vi "Auto.vi"() -> ()   [LabVIEW 2020]
uses:
  Global_Variable/Global.vi
  Global_Variable/A180648.vi
  Global_Variable/System_Conf.vi
  Libraries/S7/S7.lvlib
panel:
  out "前序":string
  out "用户事件输出":refnum<user-event>
  out "磨合正向初始化":bool
  out "工位三开始计时1":bool
  out "产品变更_Event":refnum<user-event>
  out "T1+T2":dbl
  out "T2":dbl
  out "T1":dbl
  out "吸收电流":sgl
  out "输出扭矩(大)":sgl
  out "输入扭矩":sgl
  out "力特性逆向去程":bool
  out "力特性正向去程":bool
  out "力特性逆向回程":bool
  out "力特性正向回程":bool
  out "工位三开始计时":bool
  out "工位二开始计时":bool
  out "功能正向初始化":bool
  out "功能逆向初始化":bool
  out "空载逆向初始化":bool
  out "空载正向初始化":bool
  out "试验项目":T1(tab)
  out "压装曲线":cluster{dbl[], dbl[]}[](graph)
  out "侧铆曲线":cluster{dbl[], dbl[]}[](graph)
  out "0°曲线":cluster{dbl[], dbl[]}[](graph)
  out "45°曲线":cluster{dbl[], dbl[]}[](graph)
  out "力特性试验":cluster{dbl[], dbl[]}[](graph)
  out "功能试验":cluster{dbl[], dbl[]}[](graph)
  out "电流特性试验":cluster{dbl[], dbl[]}[](graph)
  out "逆向空载试验":cluster{dbl[], dbl[]}[](graph)
  out "磨合":cluster{dbl[], dbl[]}[](graph)
  in  "判定结果":bool[][](array[boolean])=[[TRUE]]
  in  "STEP":string
  # "车速0"
  # "车速1"
  # "车速2"
  # "车速3"
  # "车速4"
  # "车速5"
  # "车速0"
  # "车速1"
  # "车速2"
  # "车速3"
  # "车速4"
  # "车速5"
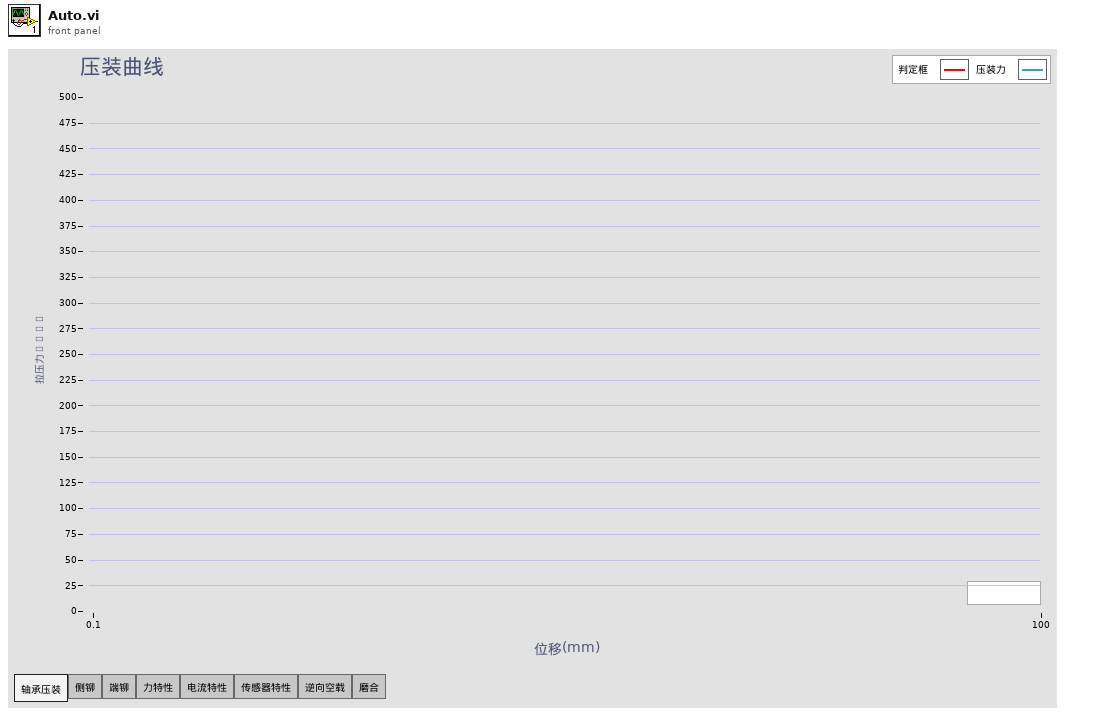
[diagram p1: front panel]
types:
  T1 = enum32{"轴承压装", "侧铆", "端铆", "力特性", "电流特性", "传感器特性", "逆向空载", "磨合"}
  T2 = enum32{"Invalid", "Standard", "Closed", "Hidden", "Minimized", "Maximized"}
  T3 = cluster{"输入轴扭矩":dbl, "输出轴扭矩小量程":dbl, "输出轴扭矩大量程":dbl}
  T4 = typedef "System_conf.ctl" = cluster{"空载滤波":bool, "逆向空载滤波":bool, "空载扭矩系数":dbl, "逆向空载扭矩系数":dbl}
  T5 = cluster{"第一段位移":cluster{"单位":string, "下限":dbl, "上限":dbl}, "第一段压力":cluster{"单位":string, "下限":dbl, "上限":dbl}, "第二段位移":cluster{"单位":string, "下限":dbl, "上限":dbl}, "第二段压力":cluster{"单位":string, "下限":dbl, "上限":dbl}}
  T6 = cluster{"第一段压力最大值":cluster{"单位":string, "下限":dbl, "上限":dbl}, "第一段压力最小值":cluster{"单位":string, "下限":dbl, "上限":dbl}, "第二段压力最大值":cluster{"单位":string, "下限":dbl, "上限":dbl}, "第二段压力最小值":cluster{"单位":string, "下限":dbl, "上限":dbl}, "最终压装位移":cluster{"单位":string, "下限":dbl, "上限":dbl}}
  T7 = typedef "lveventtype.ctl" = enum32{"Null", "Timeout", "Annotation Menu Selection", "Annotation Menu Selection?", "App Instance Close", "App Instance Close?", "Autoscale Range Change", "Bookmark Info Change", "Cell Edit", "Cell Edit?", "Cursor Grab", "Cursor Grab?", "Cursor Menu Selection", "Cursor Menu Selection?", "Cursor Move", "Cursor Release", "Data Change", "Direction Change", "Display State Change", "Drag Ended", "Drag Enter", "Drag Leave", "Drag Over", "Drag Source Update", "Drag Starting", "Drag Starting?", "Drop", "Exec State Change", "Key Down", "Key Down?", "Key Repeat", "Key Repeat?", "Key Up", "Listbox Double Click", "Menu Activation?", "Menu Selection (App)", "Menu Selection? (App)", "Menu Selection (User)", "Mouse Down", "Mouse Down?", "Mouse Enter", "Mouse Leave", "Mouse Move", "Mouse Up", "Mouse Wheel", "NI Security User Change (App)", "Pane Size", "Panel Close", "Panel Close?", "Panel Resize", "Plot Attribute Change", "Scale Range Change", "Shortcut Menu Activation?", "Shortcut Menu Selection (App)", "Shortcut Menu Selection? (App)", "Shortcut Menu Selection (User)", "Tree Double Click", "Tree Drag", "Tree Drag?", "Tree Drop", "Tree Drop?", "Tree Item Close", "Tree Item Close?", "Tree Item Open", "Tree Item Open?", "User Event", "Value Change"}
  T8 = typedef "LVPoint32TypeDef.ctl" = cluster{"Horizontal":i32, "Vertical":i32}
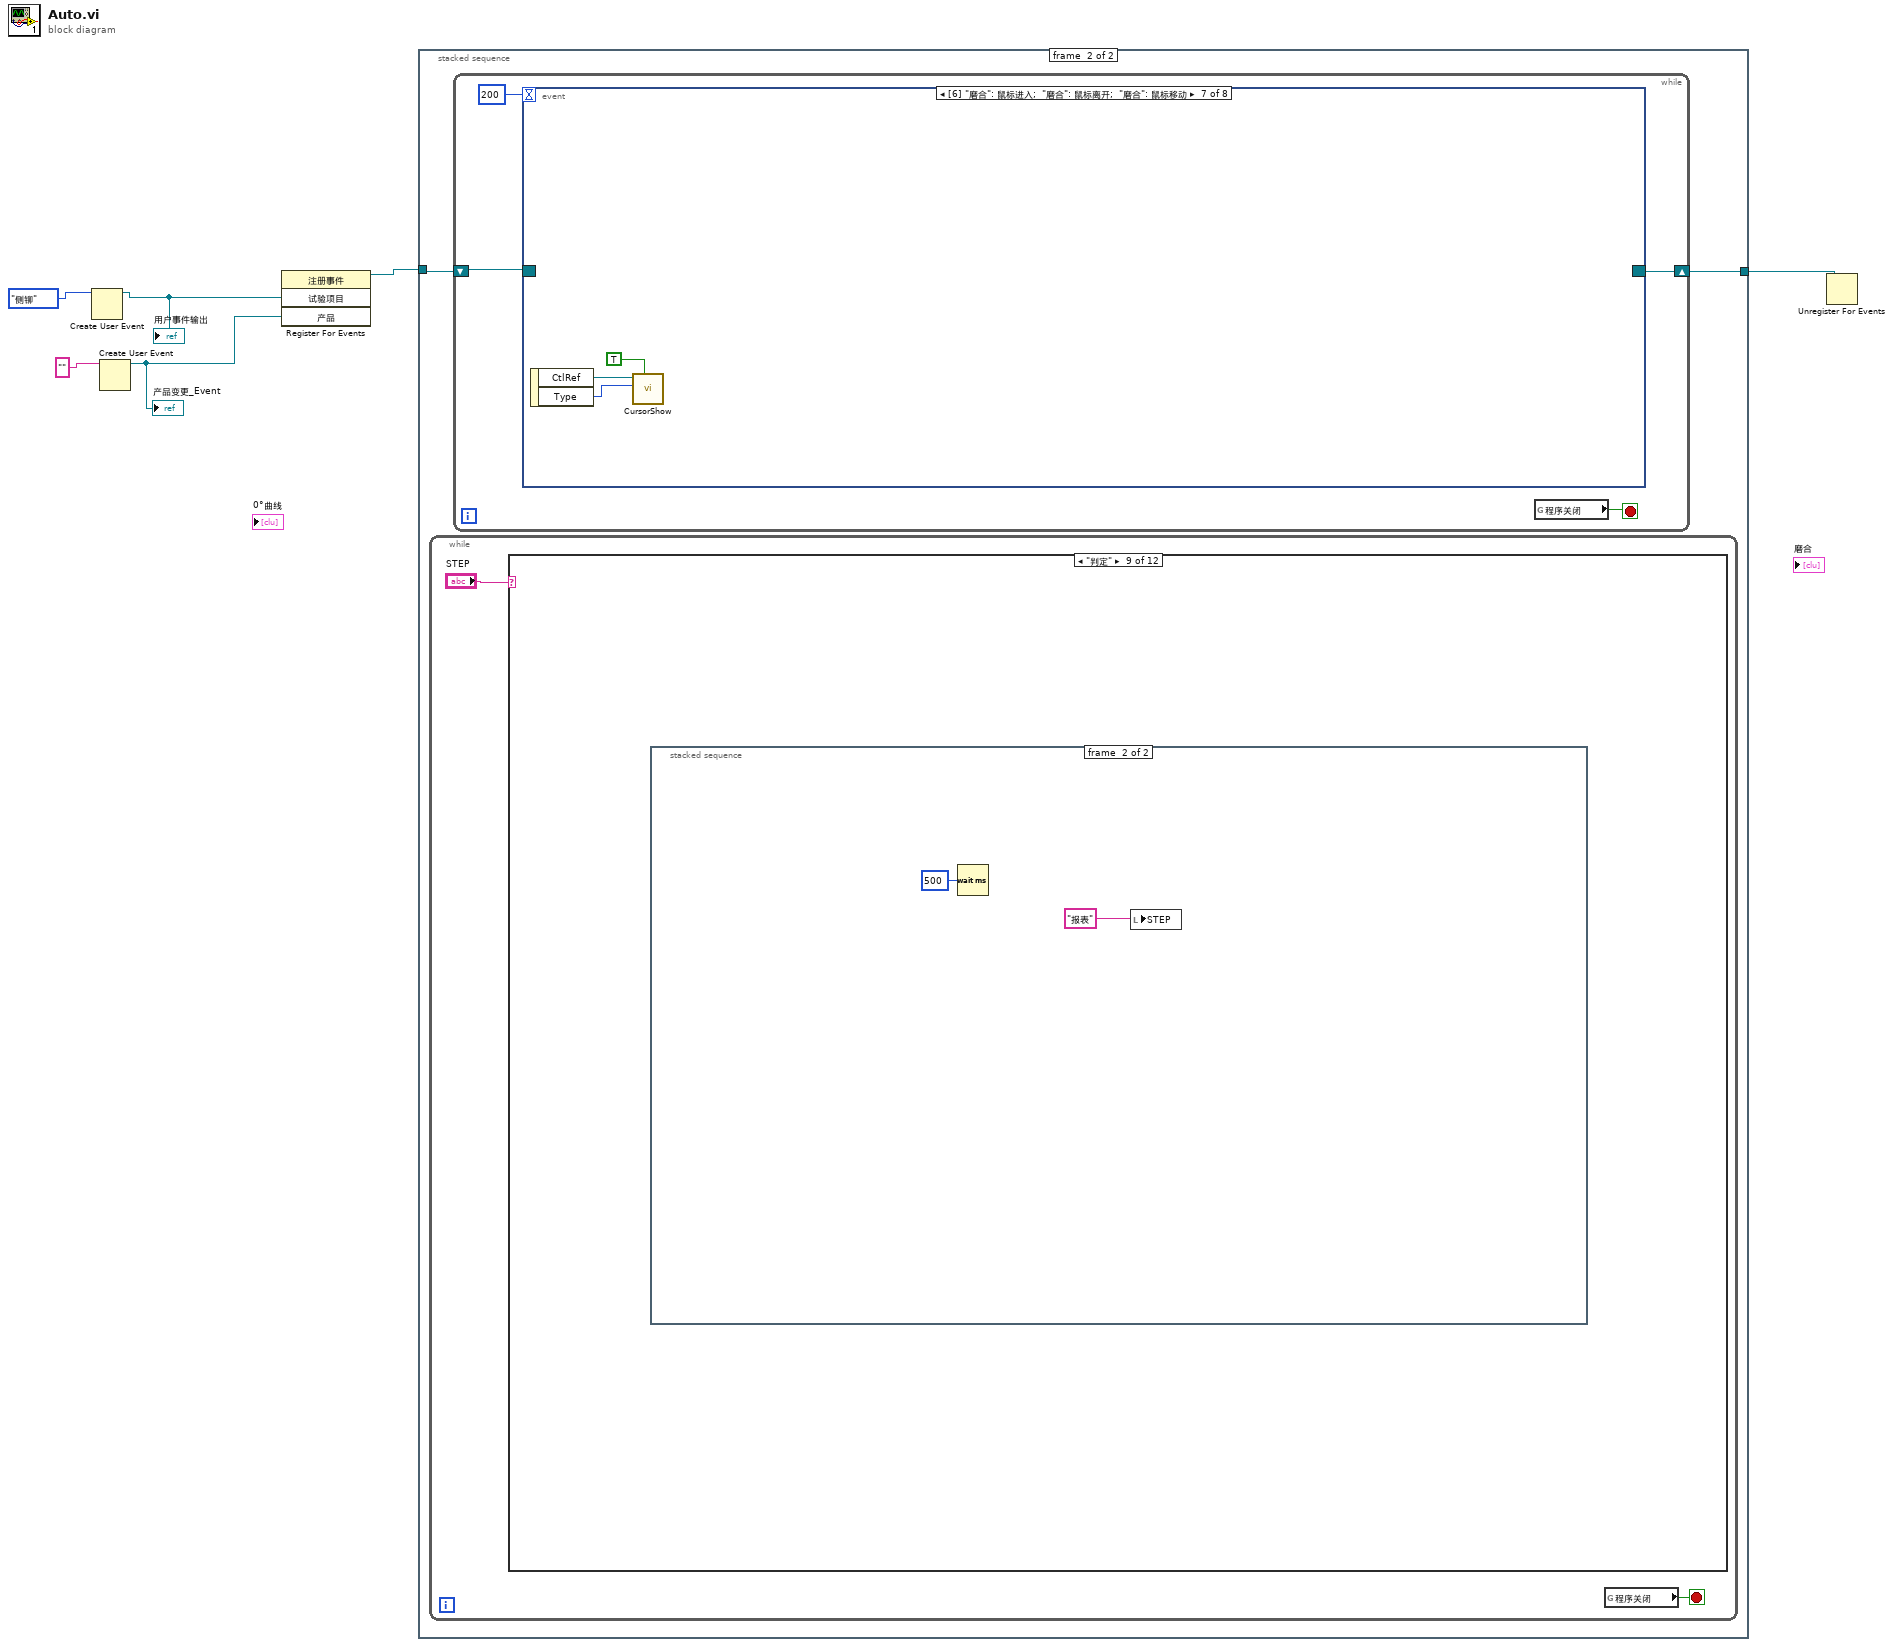
[diagram p0: block diagram]
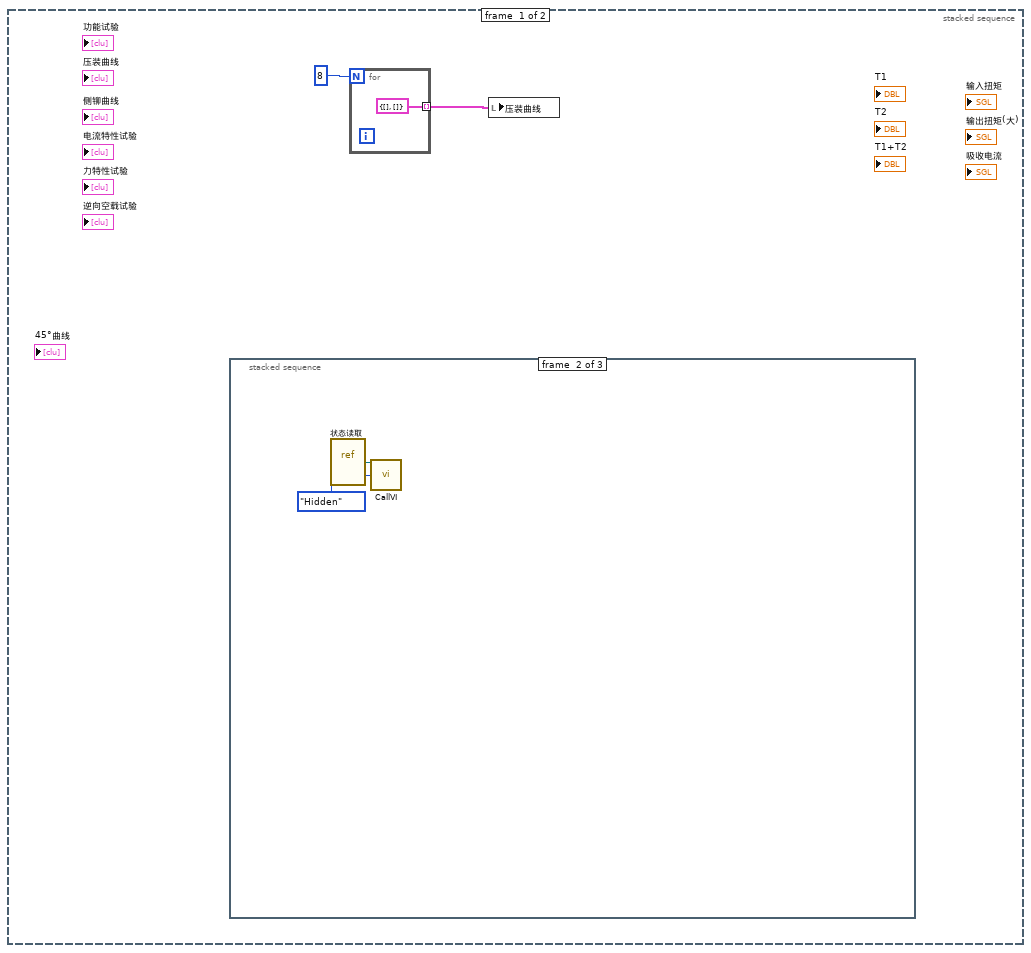
[diagram p2: hidden frame]
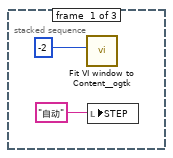
[diagram p3: hidden frame]
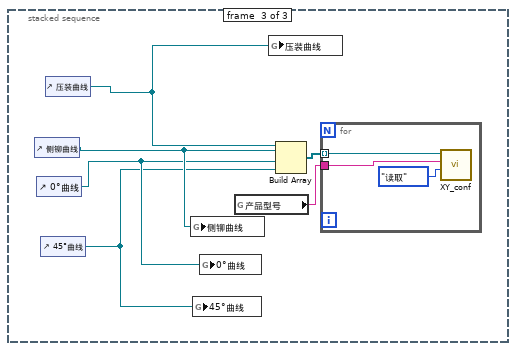
[diagram p4: hidden frame]
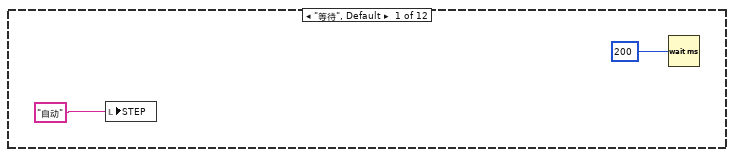
[diagram p5: hidden frame]
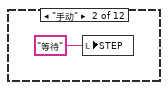
[diagram p6: hidden frame]
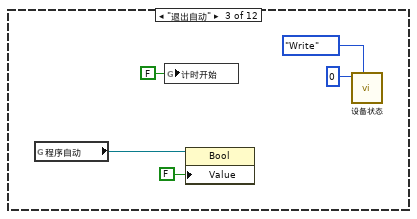
[diagram p7: hidden frame]
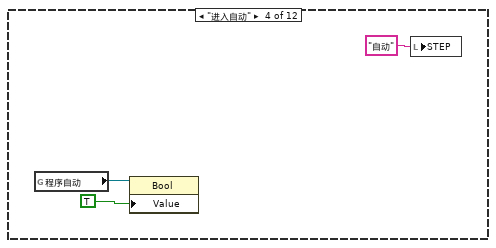
[diagram p8: hidden frame]
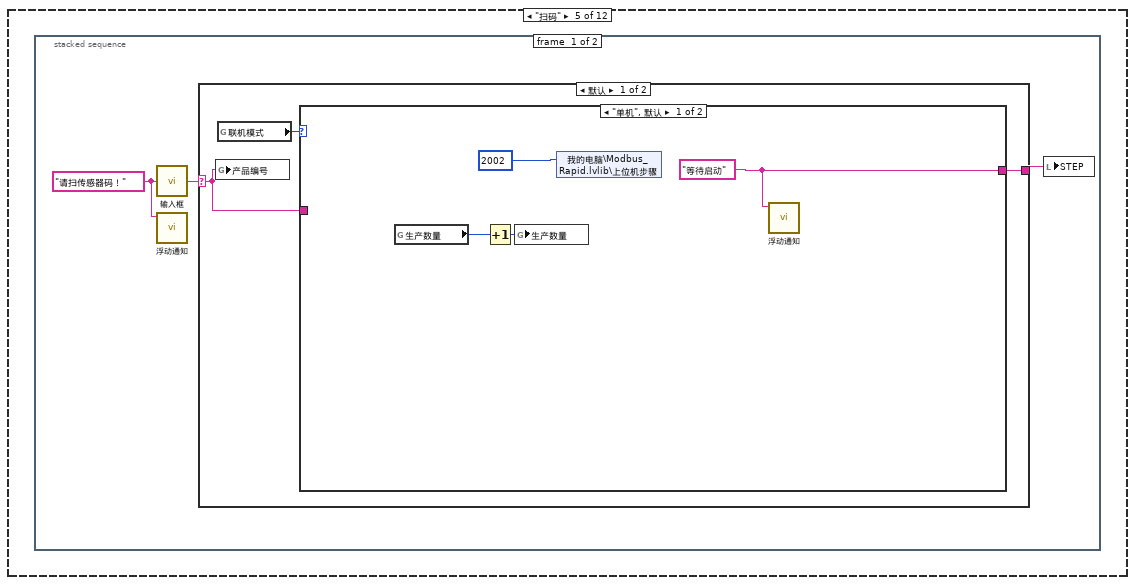
[diagram p9: hidden frame]
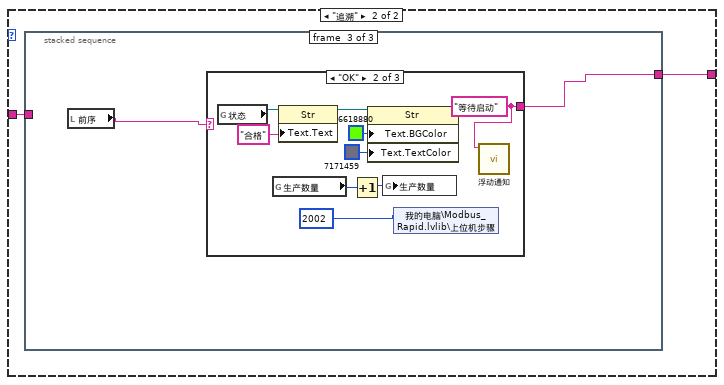
[diagram p10: hidden frame]
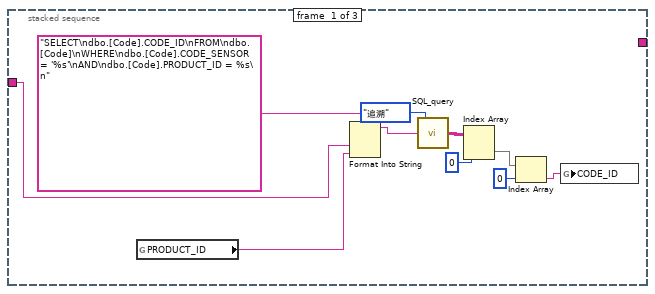
[diagram p11: hidden frame]
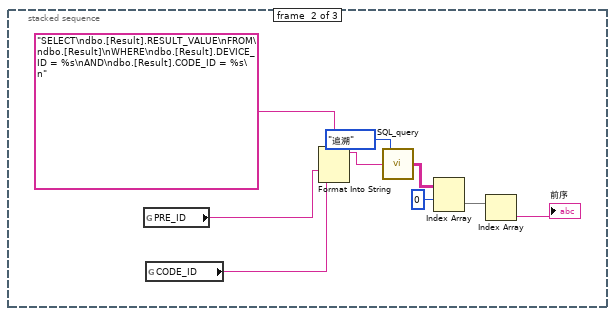
[diagram p12: hidden frame]
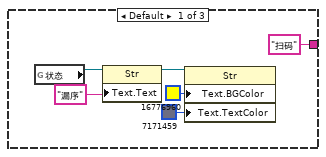
[diagram p13: hidden frame]
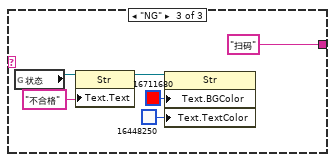
[diagram p14: hidden frame]
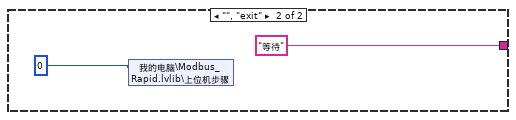
[diagram p15: hidden frame]
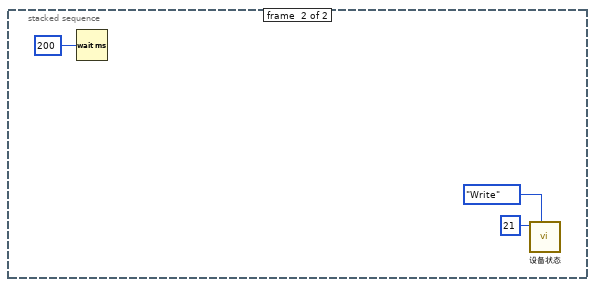
[diagram p16: hidden frame]
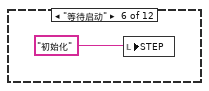
[diagram p17: hidden frame]
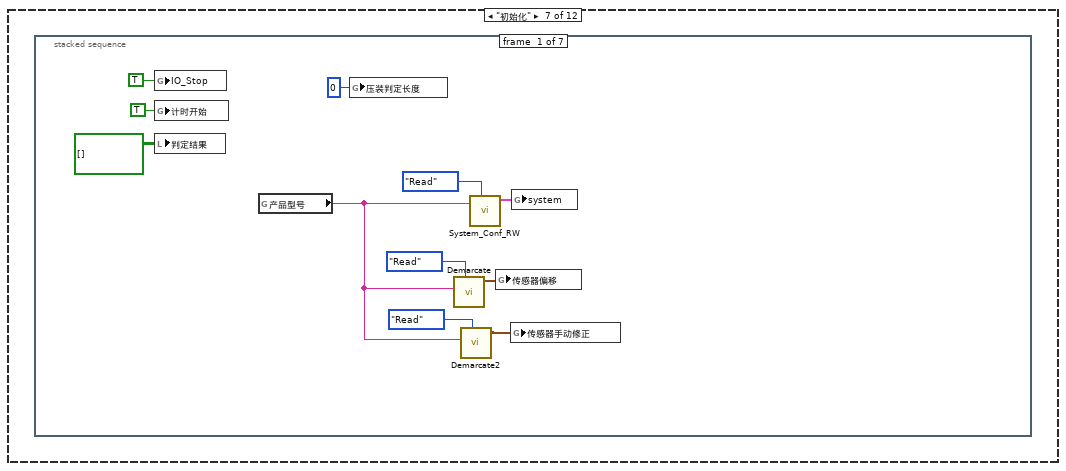
[diagram p18: hidden frame]
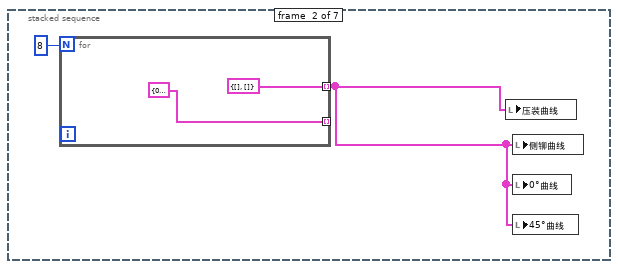
[diagram p19: hidden frame]
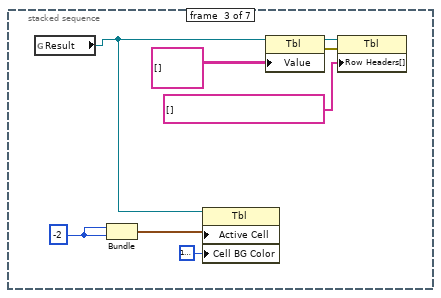
[diagram p20: hidden frame]
diagram:
  n1 = Create User Event(user event datatype=T1."侧铆" ("试验项目")) -> (user event=w1:refnum<user-event>)  [unwired: 1 in, 1 out]
  "用户事件输出" <- w1
  n2 = Create User Event(user event datatype="" ("产品")) -> (user event=w3:refnum<user-event>)  [unwired: 1 in, 1 out]
  "产品变更_Event" <- w3
  n3 = register-events(w1, w3) -> (reference out=w6:refnum<event-registration>)  [unwired: 2 in, 1 out]
  n4 = stacked-sequence {
    tunnel: w6 -> [_ w24]
    tunnel: [_ w23] -> w5
    frame #0 {
      n5 = stacked-sequence {
        frame #0 {
          n6 = call <userlib>:"Fit VI window to Content__ogtk.vi"("border spacing (2 px)"=-2) -> ()  [unwired: 5 in, 2 out]
          n7 = local write "STEP"("自动" ("STEP")) -> ()
        }
        frame #1 {
          n8 = vi-ref "状态读取.vi"() -> (w13:refnum<vi>)
          n9 = call "CallVI.vi"("VI引用"=w13, "状态"=T2."Hidden") -> ()  [unwired: 12 in, 2 out]
        }
        frame #2 {
          n10 = control-ref of="侧铆曲线"() -> (w17:refnum<vi>)
          n11 = control-ref of="0°曲线"() -> (w16:refnum<vi>)
          n12 = control-ref of="45°曲线"() -> (w15:refnum<vi>)
          n13 = control-ref of="压装曲线"() -> (w14:refnum<vi>)
          n14 = global write "A180648.vi" "侧铆曲线"(w17) -> ()
          n15 = global write "A180648.vi" "45°曲线"(w15) -> ()
          n16 = global write "A180648.vi" "0°曲线"(w16) -> ()
          n17 = global read "Global.vi" "产品型号"() -> (w18:string)
          n18 = global write "A180648.vi" "压装曲线"(w14) -> ()
          n19 = Build Array(w14, w17, w16, w15) -> (w19:refnum<vi>[])
          n20 = for {
            tunnel: w19 -> [w21] mode=indexing
            tunnel: w18 -> [w20]
            n21 = call "XY_conf.vi"("方式"=enum16{"写入", "读取"}."读取", "产品"=w20, "XY图引用"=w21) -> ()  [unwired: 4 in, 1 out]
          }
        }
      }
      n22 = for {
        N: 8 -> [_]
        tunnel: [cluster{dbl[], dbl[]} {[], []}] -> w8 mode=indexing
      }
      n23 = local write "压装曲线"(w8) -> ()
    }
    frame #1 {
      n24 = while {
        stop <- w26 stop-if-true
        n25 = case shown="\"判定\"" "STEP" {
          frame "等待", Default {
            n26 = local write "STEP"("自动" ("STEP")) -> ()
            n27 = Wait (ms)(milliseconds to wait=u32 200 ("等待时间（毫秒）")) -> ()  [unwired: 1 out]
          }
          frame "手动" {
            n28 = local write "STEP"("等待" ("STEP")) -> ()
          }
          frame "退出自动" {
            n29 = global read "Global.vi" "程序自动"() -> (w31:refnum<vi>)
            n30 = global write "Global.vi" "计时开始"(FALSE ("计时开始")) -> ()
            n31 = property class="Bool"(reference=w31, "Value"=FALSE) -> ()  [unwired: 1 in, 2 out]
            n32 = call "设备状态.vi"("枚举"=enum16{"Read", "Write"}."Write", "Status_Write"=i16 0) -> ()  [unwired: 9 in, 1 out]
          }
          frame "进入自动" {
            n33 = global read "Global.vi" "程序自动"() -> (w36:refnum<vi>)
            n34 = property class="Bool"(reference=w36, "Value"=TRUE) -> ()  [unwired: 1 in, 2 out]
            n35 = local write "STEP"("自动" ("STEP")) -> ()
          }
          frame "扫码" {
            n36 = stacked-sequence {
              frame #0 {
                w39 = "请扫传感器码！" ("提示信息")
                n37 = call "输入框.vi"("提示信息"=w39) -> ("条形码输出"=w40:string)
                n38 = call "浮动通知.vi"("通知内容"=w39) -> ()  [unwired: 11 in]
                n39 = case shown="默认" w40 {
                  selector: w40 -> [w41 _]
                  tunnel: [w43 "等待" ("State(s) in Front (\"\")")] -> w38
                  frame Default {
                    n40 = global write "Global.vi" "产品编号"(w41) -> ()
                    n41 = global read "Global.vi" "联机模式"() -> (w42:enum16{"单机", "追溯"})
                    n42 = case shown="\"单机\", 默认" w42 {
                      tunnel: [w45 w49] -> w43
                      tunnel: w41 -> [_ w48]
                      frame "单机", Default {
                        w45 = "等待启动" ("State(s) in Front (\"\")")
                        n43 = global read "Global.vi" "生产数量"() -> (w46:i32)
                        n44 = Increment(x=w46) -> (x+1=w47:i32)
                        n45 = global write "Global.vi" "生产数量"(w47) -> ()
                        n46 = shared-variable "我的电脑\\Modbus_Rapid.lvlib\\上位机步骤"(u16 2002 ("设备状态")) -> ()  [unwired: 1 in, 1 out]
                        n47 = call "浮动通知.vi"("通知内容"=w45) -> ()  [unwired: 11 in]
                      }
                      frame "追溯" {
                        n48 = stacked-sequence {
                          tunnel: [_ _ w70] -> w49
                          tunnel: w48 -> [w58 _ _]
                          frame #0 {
                            n49 = global read "追溯Global.vi" "PRODUCT_ID"() -> (w57:string)
                            n50 = Format Into String(format string="SELECT\ndbo.[Code].CODE_ID\nFROM\ndbo.[Code]\nWHERE\ndbo.[Code].CODE_SENSOR = '%s'\nAND\ndbo.[Code].PRODUCT_ID = %s\n" ("格式字符串"), w58, w57) -> (resulting string=w56:string)  [unwired: 2 in, 1 out]
                            n51 = call "SQL_query.vi"("SQL query"=w56, "联机模式"=enum16{"单机", "追溯"}."追溯") -> ("data"=w54:string[][])  [unwired: 2 in, 1 out]
                            n52 = Index Array(array=w54, index (row)=0 ("索引 (行)")) -> (element=w52:string[])  [unwired: 1 in]
                            n53 = Index Array(array=w52, index=0 ("索引")) -> (element=w50:string)
                            n54 = global write "追溯Global.vi" "CODE_ID"(w50) -> ()
                          }
                          frame #1 {
                            n55 = global read "追溯Global.vi" "PRE_ID"() -> (w67:string)
                            n56 = global read "追溯Global.vi" "CODE_ID"() -> (w66:string)
                            n57 = Format Into String(format string="SELECT\ndbo.[Result].RESULT_VALUE\nFROM\ndbo.[Result]\nWHERE\ndbo.[Result].DEVICE_ID = %s\nAND\ndbo.[Result].CODE_ID = %s\n" ("格式字符串"), w67, w66) -> (resulting string=w65:string)  [unwired: 2 in, 1 out]
                            n58 = call "SQL_query.vi"("SQL query"=w65, "联机模式"=enum16{"单机", "追溯"}."追溯") -> ("data"=w63:string[][])  [unwired: 2 in, 1 out]
                            n59 = Index Array(array=w63, index (row)=0 ("索引 (行)")) -> (element=w61:string[])  [unwired: 1 in]
                            n60 = Index Array(array=w61) -> (element=→"前序":string)  [unwired: 1 in]
                          }
                          frame #2 {
                            n61 = local read "前序"() -> (w69:string)
                            n62 = case shown="\"OK\"" w69 {
                              tunnel: ["扫码" ("State(s) in Front (\"\")") w80 "扫码" ("State(s) in Front (\"\")")] -> w70
                              frame Default {
                                n63 = global read "Global.vi" "状态"() -> (w76:refnum<vi>)
                                n64 = property class="Str"(reference=w76, "Text.Text"="漏序" ("文本.文本")) -> (reference out=w75:refnum<vi>)  [unwired: 1 in, 1 out]
                                n65 = property class="Str"(reference=w75, "Text.BGColor"=u32 16776960 ("文本.文本颜色:背景色"), "Text.TextColor"=u32 7171459 ("文本.文本颜色:文本颜色")) -> ()  [unwired: 1 in, 2 out]
                              }
                              frame "OK" {
                                w80 = "等待启动" ("State(s) in Front (\"\")")
                                n66 = global read "Global.vi" "状态"() -> (w85:refnum<vi>)
                                n67 = global read "Global.vi" "生产数量"() -> (w78:i32)
                                n68 = property class="Str"(reference=w85, "Text.Text"="合格" ("文本.文本")) -> (reference out=w83:refnum<vi>)  [unwired: 1 in, 1 out]
                                n69 = Increment(x=w78) -> (x+1=w79:i32)
                                n70 = property class="Str"(reference=w83, "Text.BGColor"=u32 6618880 ("文本.文本颜色:背景色"), "Text.TextColor"=u32 7171459 ("文本.文本颜色:文本颜色")) -> ()  [unwired: 1 in, 2 out]
                                n71 = global write "Global.vi" "生产数量"(w79) -> ()
                                n72 = shared-variable "我的电脑\\Modbus_Rapid.lvlib\\上位机步骤"(u16 2002 ("设备状态")) -> ()  [unwired: 1 in, 1 out]
                                n73 = call "浮动通知.vi"("通知内容"=w80) -> ()  [unwired: 11 in]
                              }
                              frame "NG" {
                                n74 = global read "Global.vi" "状态"() -> (w91:refnum<vi>)
                                n75 = property class="Str"(reference=w91, "Text.Text"="不合格" ("文本.文本")) -> (reference out=w89:refnum<vi>)  [unwired: 1 in, 1 out]
                                n76 = property class="Str"(reference=w89, "Text.BGColor"=u32 16711680 ("文本.文本颜色:背景色"), "Text.TextColor"=u32 16448250 ("文本.文本颜色:文本颜色")) -> ()  [unwired: 1 in, 2 out]
                              }
                            }
                          }
                        }
                      }
                    }
                  }
                  frame "", "exit" {
                    n77 = shared-variable "我的电脑\\Modbus_Rapid.lvlib\\上位机步骤"(u16 0 ("设备状态")) -> ()  [unwired: 1 in, 1 out]
                  }
                }
                n78 = local write "STEP"(w38) -> ()
              }
              frame #1 {
                n79 = Wait (ms)(milliseconds to wait=u32 200 ("等待时间（毫秒）")) -> ()  [unwired: 1 out]
                n80 = call "设备状态.vi"("枚举"=enum16{"Read", "Write"}."Write", "Status_Write"=i16 21) -> ()  [unwired: 9 in, 1 out]
              }
            }
          }
          frame "等待启动" {
            n81 = local write "STEP"("初始化" ("STEP")) -> ()
          }
          frame "初始化" {
            n82 = stacked-sequence {
              frame #0 {
                n83 = global write "Global.vi" "IO_Stop"(TRUE ("IO_Stop")) -> ()
                n84 = global write "Global.vi" "计时开始"(TRUE ("计时开始")) -> ()
                n85 = local write "判定结果"(bool[][] [] ("判定结果")) -> ()
                n86 = global read "Global.vi" "产品型号"() -> (w99:string)
                n87 = global write "判定参数.vi" "压装判定长度"(0 ("拉轴判定长度")) -> ()
                n88 = call "Demarcate.vi"("Mode"=enum16{"Read", "Write"}."Read", "Section"=w99) -> ("Sensor OUT"=w103:T3)  [unwired: 8 in, 1 out]
                n89 = call "Demarcate2.vi"("Mode"=enum16{"Read", "Write"}."Read", "Section"=w99) -> ("Sensor OUT"=w102:T3)  [unwired: 8 in, 1 out]
                n90 = call "System_Conf_RW.vi"("Mode"=enum16{"Read", "Write"}."Read", "Section"=w99) -> ("system_out"=w105:T4)  [unwired: 8 in, 1 out]
                n91 = global write "传感器偏移.vi" "传感器偏移"(w103) -> ()
                n92 = global write "传感器偏移.vi" "传感器手动修正"(w102) -> ()
                n93 = global write "System_Conf.vi" "system"(w105) -> ()
              }
              frame #1 {
                n94 = for {
                  N: 8 -> [_]
                  tunnel: [cluster{dbl[], dbl[]} {[], []}] -> w109 mode=indexing
                  tunnel: [cluster{"f0":dbl, "df":dbl, "magnitude":dbl[]} {"f0"=0.0, "df"=0.0, "magnitude"=[]} ("power spectrum [dB EU]")] -> _ mode=indexing
                }
                n95 = local write "压装曲线"(w109) -> ()
                n96 = local write "侧铆曲线"(w109) -> ()
                n97 = local write "0°曲线"(w109) -> ()
                n98 = local write "45°曲线"(w109) -> ()
              }
              frame #2 {
                w114 = -2
                n99 = global read "Global.vi" "Result"() -> (w116:refnum<vi>)
                n100 = Bundle(w114, w114) -> (w113:cluster{i32, i32})  [unwired: 1 in]
                n101 = property class="Tbl"(reference=w116, "Active Cell"=w113, "Cell BG Color"=u32 16777216 ("活动单元格:单元格背景色")) -> ()  [unwired: 1 in, 2 out]
                n102 = property class="Tbl"(reference=w116, "Value"=string[][] []) -> (reference out=w119:refnum<vi>, error out=w120:errorcluster)  [unwired: 1 in]
                n103 = property class="Tbl"(reference=w119, error in=w120, "Row Headers[]"=string[] [] ("列首字符串[]")) -> ()  [unwired: 2 out]
              }
              frame #3 {
                n104 = global read "A180648.vi" "LED-轴承压装"() -> (w124:refnum<vi>)
                n105 = global read "A180648.vi" "LED-端铆"() -> (w121:refnum<vi>)
                n106 = global read "A180648.vi" "LED-侧铆"() -> (w122:refnum<vi>)
                n107 = Build Array(w124, w122, w121) -> (w123:refnum<vi>[])
                n108 = for {
                  tunnel: w123 -> [w125] mode=indexing
                  n109 = property class="Bool"(reference=w125, "Colors [4]"=cluster{u32, u32}[] [{12369084, 12369084}] ("颜色[4]")) -> ()  [unwired: 1 in, 2 out]
                }
              }
              frame #4 {
                w128 = 1 ("维数大小")
                n110 = Initialize Array(" " ("字符串"), w128, w128, w128) -> (w130:string[][][])
                n111 = global write "A180648.vi" "当前检测项"(enum32{"拉轴", "卡簧", "完成"}."拉轴" ("当前检测项")) -> ()
                n112 = global write "A180648.vi" "检测结果"(w130) -> ()
              }
              frame #5 {
                n113 = local read "压装曲线"() -> (w132:cluster{dbl[], dbl[]}[])
                n114 = global read "判定参数.vi" "判定框"() -> (w133:T5)
                n115 = for {
                  tunnel: w132 -> [w136] mode=indexing
                  tunnel: [w135] -> w131 mode=indexing
                  tunnel: w133 -> [w134]
                  i -> [w137]
                  n116 = case shown="0" w137 {
                    tunnel: w136 -> [w138 _]
                    tunnel: [w138 w141] -> w135
                    tunnel: w134 -> [_ w146]
                    frame Default {
                    }
                    frame 0 {
                      n117 = Unbundle By Name(w146) -> ("第一段位移.下限"=w145:dbl, "第一段位移.上限"=w144:dbl, "第一段压力.下限"=w139:dbl, "第一段压力.上限"=w140:dbl)
                      n118 = Build Array(w144, w144, w145, w145, w144) -> (w143:dbl[])
                      n119 = Build Array(w139, w140, w140, w139, w139) -> (w142:dbl[])
                      n120 = Bundle(w143, w142) -> (w141:cluster{dbl[], dbl[]})  [unwired: 1 in]
                    }
                  }
                }
                n121 = local write "压装曲线"(w131) -> ()
              }
              frame #6 {
                w148 = TRUE
                n122 = local write "STEP"("自动" ("STEP")) -> ()
                "工位三开始计时" <- w148
                "工位二开始计时" <- w148
                "空载正向初始化" <- w148
                "空载逆向初始化" <- w148
                "功能正向初始化" <- w148
                "功能逆向初始化" <- w148
                "力特性逆向去程" <- w148
                "力特性正向去程" <- w148
                "力特性逆向回程" <- w148
                "力特性正向回程" <- w148
                "磨合正向初始化" <- w148
                "工位三开始计时1" <- w148
              }
            }
          }
          frame "试验项" {
            n123 = global read "A180648.vi" "当前检测项"() -> (w149:enum32{"拉轴", "卡簧", "完成"})
            n124 = case shown="\"拉轴\", 默认" w149 {
              selector: w149 -> [w151 _]
              tunnel: [w154 "报表" ("STEP")] -> w150
              frame "拉轴", Default {
                n125 = global read "Global.vi" "试验项目"() -> (w152:bool[])
                n126 = Index Array(array=w152, index=w151) -> (element=w153:bool)
                n127 = case shown="真" w153 {
                  tunnel: ["试验项" ("字符串") w161] -> w154
                  tunnel: w151 -> [_ w162]
                  frame False {
                    n128 = global read "A180648.vi" "当前检测项"() -> (w159:enum32{"拉轴", "卡簧", "完成"})
                    n129 = Increment(x=w159) -> (x+1=w158:enum32{"拉轴", "卡簧", "完成"})
                    n130 = global write "A180648.vi" "当前检测项"(w158) -> ()
                    n131 = local read "判定结果"() -> (w155:bool[][])
                    n132 = Build Array (concatenate)(w155, bool[] [FALSE] ("判定结果")) -> (w156:bool[][])
                    n133 = local write "判定结果"(w156) -> ()
                  }
                  frame True {
                    n134 = case shown="\"拉轴\", 默认" w162 {
                      tunnel: ["等待" ("STEP") "等待" ("STEP") "报表" ("STEP")] -> w161
                      frame "拉轴", Default {
                        n135 = call "浮动通知.vi"("通知内容"="拉拔力试验") -> ()  [unwired: 11 in]
                        n136 = property on="试验项目" class="TabCtl (严格)"("Val(Sgnl)"=T1."轴承压装" ("值(信号)")) -> ()  [unwired: 2 in, 2 out]
                      }
                      frame "卡簧" {
                        n137 = call "浮动通知.vi"("通知内容"="卡簧检测") -> ()  [unwired: 11 in]
                      }
                      frame "完成" {
                      }
                    }
                  }
                }
              }
              frame "完成" {
              }
            }
            n138 = local write "STEP"(w150) -> ()
          }
          frame "判定" {
            n139 = stacked-sequence {
              frame #0 {
                n140 = global read "判定参数.vi" "压装判定参数"() -> (w181:T6)
                n141 = local read "压装曲线"() -> (w182:cluster{dbl[], dbl[]}[])
                n142 = global read "Global.vi" "Result"() -> (w180:refnum<vi>)
                n143 = call "压装试验判定.vi"("Result"=w180, "判定参数"=w181, "XY曲线"=w182) -> ("判定项长度"=w171:i32, "OK？"=w170:bool)  [unwired: 7 in]
                n144 = global read "A180648.vi" "LED-轴承压装"() -> (w176:refnum<vi>)
                n145 = local read "判定结果"() -> (w172:bool[][])
                n146 = Select(t=cluster{u32, u32}[] [{6618880, 6618880}, {6618880, 6618880}, {6618880, 6618880}, {6618880, 6618880}] ("颜色[4]"), s=w170, f=cluster{u32, u32}[] [{16711680, 16711680}, {16711680, 16711680}, {16711680, 16711680}, {16711680, 16711680}] ("颜色[4]")) -> (s? t:f=w177:cluster{u32, u32}[])
                n147 = Build Array(TRUE, w170) -> (w175:bool[])
                n148 = global write "判定参数.vi" "压装判定长度"(w171) -> ()
                n149 = property class="Bool"(reference=w176, "Colors [4]"=w177) -> ()  [unwired: 1 in, 2 out]
                n150 = Build Array (concatenate)(w172, w175) -> (w173:bool[][])
                n151 = case shown="真" w170 {
                  frame False {
                    n152 = shared-variable "我的电脑\\Modbus_Rapid.lvlib\\工位1合格状态"(u16 2 ("工位1合格状态")) -> ()  [unwired: 1 in, 1 out]
                  }
                  frame True {
                    n153 = shared-variable "我的电脑\\Modbus_Rapid.lvlib\\工位1合格状态"(u16 1 ("工位1合格状态")) -> ()  [unwired: 1 in, 1 out]
                  }
                }
                n154 = local write "判定结果"(w173) -> ()
              }
              frame #1 {
                n155 = Wait (ms)(milliseconds to wait=u32 500 ("等待时间（毫秒）")) -> ()  [unwired: 1 out]
                n156 = local write "STEP"("报表") -> ()
              }
            }
          }
          frame "自动" {
            n157 = shared-variable "我的电脑\\Modbus_Rapid.lvlib\\上位机步骤"() -> (w187:u16)  [unwired: 1 in, 1 out]
            n158 = case shown="10" w187 {
              frame 127 {
                n159 = global write "Global.vi" "计时开始"(FALSE ("计时开始")) -> ()
                n160 = call "浮动通知.vi"("通知内容"="复位中……" ("Status")) -> ()  [unwired: 11 in]
              }
              frame 128 {
                n161 = call "浮动通知.vi"("通知内容"="复位完成" ("Status")) -> ()  [unwired: 11 in]
              }
              frame Default {
              }
              frame 0 {
                n162 = disable-structure shown="禁用" {
                  frame Disabled {
                    n163 = global write "Global.vi" "计时开始"(FALSE ("计时开始")) -> ()
                  }
                  frame Enabled {
                  }
                }
              }
              frame 2 {
                n164 = local write "STEP"("初始化" ("STEP")) -> ()
              }
              frame 5 {
                n165 = shared-variable "我的电脑\\Modbus_Rapid.lvlib\\上位机步骤"(u16 10 ("上位机状态")) -> ()  [unwired: 1 in, 1 out]
              }
              frame 7 {
                n166 = shared-variable "我的电脑\\Modbus_Rapid.lvlib\\电缸参数"() -> (w197:sgl[])  [unwired: 1 in, 1 out]
                n167 = disable-structure shown="禁用" {
                  frame Disabled {
                    n168 = local read "压装曲线"() -> (w200:cluster{dbl[], dbl[]}[])
                    n169 = for {
                      tunnel: [w202] -> _ mode=indexing
                      tunnel: w200 -> [w201] mode=indexing
                      i -> [w203]
                      n170 = case shown="2" w203 {
                        tunnel: [_ w204] -> w202
                        tunnel: w201 -> [_ w209]
                        frame Default {
                        }
                        frame 2 {
                          n171 = Unbundle(w209) -> (w208:dbl[], w207:dbl[])
                          n172 = Build Array(w208) -> (w206:dbl[][])  [unwired: 1 in]
                          n173 = Build Array(w207) -> (w205:dbl[][])  [unwired: 1 in]
                          n174 = Bundle(w206, w205) -> (w204:cluster{dbl[][], dbl[][]})  [unwired: 1 in]
                        }
                      }
                    }
                    n175 = local read "压装曲线"() -> ()  [unwired: 1 in]
                  }
                  frame Enabled {
                  }
                }
                n176 = Index Array(array=w197, index=1 ("索引")) -> (element=w196:sgl)
                n177 = Index Array(array=w197) -> (element=w195:sgl)  [unwired: 1 in]
                n178 = control-ref of="压装曲线"() -> (w199:refnum<vi>)
                n179 = call "曲线采集.vi"("曲线引用"=w199, "曲线索引"=2, "X"=w196, "Y"=w195) -> ()  [unwired: 10 in, 2 out]
              }
              frame 8 {
                n180 = call "浮动通知.vi"("通知内容"="程序停止！" ("Status")) -> ()  [unwired: 11 in]
              }
              frame 10 {
                n181 = local write "STEP"("判定" ("STEP")) -> ()
              }
              frame 20 {
                n182 = shared-variable "我的电脑\\Modbus_Rapid.lvlib\\上位机步骤"() -> (w212:u16)  [unwired: 1 in, 1 out]
                n183 = case shown="2000" w212 {
                  frame 0, Default {
                  }
                  frame 2000 {
                    n184 = local write "STEP"("扫码" ("STEP")) -> ()
                  }
                }
              }
              frame 100 {
                n185 = call "浮动通知.vi"("通知内容"="请安装工件到位启动！" ("Status")) -> ()  [unwired: 11 in]
              }
              frame 105 {
                n186 = call "浮动通知.vi"("通知内容"="压紧缸下降！" ("Status")) -> ()  [unwired: 11 in]
              }
              frame 120 {
                n187 = call "浮动通知.vi"("通知内容"="夹爪夹紧！" ("Status")) -> ()  [unwired: 11 in]
              }
              frame 130 {
                n188 = call "浮动通知.vi"("通知内容"="拉升磨合" ("Status")) -> ()  [unwired: 11 in]
              }
              frame 161 {
                n189 = call "浮动通知.vi"("通知内容"="夹爪松开" ("Status")) -> ()  [unwired: 11 in]
                n190 = local write "STEP"("判定" ("STEP")) -> ()
              }
              frame 163 {
                n191 = call "浮动通知.vi"("通知内容"="请取记号笔" ("Status")) -> ()  [unwired: 11 in]
              }
              frame 999 {
                n192 = call "浮动通知.vi"("通知内容"="请启动！" ("Status")) -> ()  [unwired: 11 in]
              }
              frame 2000 {
                n193 = shared-variable "我的电脑\\Modbus_Rapid.lvlib\\上位机步骤"(u16 2001 ("上位机步骤")) -> ()  [unwired: 1 in, 1 out]
                n194 = local write "STEP"("扫码" ("STEP")) -> ()
              }
              frame 1002 {
              }
              frame 1024 {
                n195 = local write "STEP"("退出自动" ("STEP")) -> ()
              }
            }
          }
          frame "合格判定" {
            n196 = Wait (ms)(milliseconds to wait=u32 100 ("等待时间（毫秒）")) -> ()  [unwired: 1 out]
            n197 = local write "STEP"("等待" ("STEP")) -> ()
          }
          frame "报表" {
            n198 = stacked-sequence {
              seq-local: [_ w231 _ _] -> [_ _ w236 _]
              frame #0 {
                n199 = global write "Global.vi" "计时开始"(FALSE ("计时开始")) -> ()
                n200 = disable-structure shown="禁用" {
                  frame Disabled {
                    n201 = global read "Global.vi" "产品编号"() -> (w230:string)
                    n202 = call "Get_CODE_ID.vi"("CODE_MAIN"=w230) -> ("CODE_ID"=w229:string)  [unwired: 10 in]
                    n203 = global write "追溯Global.vi" "CODE_ID"(w229) -> ()
                  }
                  frame Enabled {
                  }
                }
                n204 = shared-variable "我的电脑\\Modbus_Rapid.lvlib\\上位机步骤"(u16 1000 ("上位机状态")) -> ()  [unwired: 1 in, 1 out]
              }
              frame #1 {
                n205 = global read "Global.vi" "产品编号"() -> (w232:string)
                n206 = call "Report.vi"("文件重命名"=TRUE, "文件名称"=w232, "检测结果"="判定结果") -> ("PRODUCT_VAULE"=w231:string)  [unwired: 7 in, 1 out]
              }
              frame #2 {
                n207 = global read "Global.vi" "联机模式"() -> (w235:enum16{"单机", "追溯"})
                n208 = case shown="\"追溯\"" w235 {
                  tunnel: w236 -> [_ w237]
                  frame "单机", Default {
                  }
                  frame "追溯" {
                    n209 = global read "Global.vi" "Result"() -> (w239:refnum<vi>)
                    n210 = property class="Tbl"(reference=w239) -> (reference out=w244:refnum<vi>, error out=w241:errorcluster, "Row Headers[]"=w242:string[])  [unwired: 1 in]
                    n211 = property class="Tbl"(reference=w244, error in=w241) -> (error out=w240:errorcluster, "Value"=w243:string[][])  [unwired: 1 out]
                    n212 = for {
                      tunnel: w243 -> [w251] mode=indexing
                      tunnel: w242 -> [w252] mode=indexing
                      tunnel: [w249] -> w238 mode=indexing if=w250
                      shift-right: [w248] -> _
                      shift-left: w240 -> [w248]
                      n213 = Build Array (concatenate)(w252, w251) -> (w249:string[])
                      n214 = Index Array(array=w251) -> (element=w253:string)  [unwired: 1 in]
                      n215 = case shown="\"\"" w253 {
                        tunnel: [TRUE FALSE] -> w250
                        frame Default {
                        }
                        frame "" {
                        }
                      }
                    }
                    n216 = global read "追溯Global.vi" "DEVICE_ID"() -> (w246:string)
                    n217 = global read "追溯Global.vi" "CODE_ID"() -> (w247:string)
                    n218 = global read "追溯Global.vi" "USER_ID"() -> (w245:string)
                    n219 = call "UPTEST.vi"("Result"=w238, "CODE_ID"=w247, "DEVICE_ID"=w246) -> ()  [unwired: 6 in, 1 out]
                    n220 = call "UPRESULT.vi"("DEVICE_ID"=w246, "USER_ID"=w245, "CODE_ID"=w247, "RESULT_VALUE"=w237) -> ()  [unwired: 11 in, 1 out]
                  }
                }
              }
              frame #3 {
                n221 = global read "检测结果.vi" "合格状态"() -> (w257:string)
                n222 = local write "STEP"("进入自动" ("STEP")) -> ()
                n223 = case shown="\"假\", 默认" w257 {
                  frame "假", Default {
                  }
                  frame "合格" {
                    n224 = global read "Global.vi" "合格数量"() -> (w260:i32)
                    n225 = Increment(x=w260) -> (x+1=w259:i32)
                    n226 = global write "Global.vi" "合格数量"(w259) -> ()
                  }
                }
                n227 = Wait (ms)(milliseconds to wait=u32 1000 ("等待时间（毫秒）")) -> ()  [unwired: 1 out]
              }
            }
          }
        }
        n228 = global read "Global.vi" "程序关闭"() -> (w26:bool)
      }
      n229 = while {
        shift-right: [w261] -> w23
        shift-left: w24 -> [w262]
        stop <- w263 stop-if-true
        n230 = event shown="[6] \"磨合\": 鼠标进入;  \"磨合\": 鼠标离开;  \"磨合\": 鼠标移动" {
          selector: w262 -> [_ _ _ _ _ _ _ _]
          dyn-events: [_ _ _ _ _ _ _ _] -> w261
          timeout: 200 -> [_ _ _ _ _ _ _ _]
          event Timeout {
            n231 = event-data() -> ()  [unwired: 1 in, 3 out]
            n232 = call "Obtain Broadcast Events for Registration.vi"() -> ("Already running?"=w265:bool)  [unwired: 9 in, 2 out]
            n233 = case shown="真" w265 {
              frame False {
                n234 = local write "STEP"("手动" ("STEP")) -> ()
              }
              frame True {
                n235 = call "错误代码.vi"() -> ("Status_Read"=w267:u32)  [unwired: 11 in]
                n236 = feedback #1() -> (w277:u32)  [unwired: 1 in]
                n237 = feedback-in #1(w267) -> ()
                n238 = case shown="0" w267 {
                  frame 0 {
                    n239 = global read "Global.vi" "报警图标"() -> (w278:refnum<vi>)
                    n240 = property class="Bool"(reference=w278, "Visible"=FALSE ("可见")) -> ()  [unwired: 1 in, 2 out]
                  }
                  frame 1, Default {
                    n241 = global read "Global.vi" "报警图标"() -> (w281:refnum<vi>)
                    n242 = property class="Bool"(reference=w281, "Visible"=TRUE ("可见")) -> ()  [unwired: 1 in, 2 out]
                  }
                }
                n243 = Greater Or Equal?(x=w267, y=i16 5000) -> (x >= y?=w275:bool)
                n244 = Less?(x=w267, y=i16 5200) -> (x < y?=w276:bool)
                n245 = Equal?(x=w267, y=w277) -> (x = y?=w274:bool)
                n246 = global read "Global.vi" "报警图标"() -> (w269:refnum<vi>)
                n247 = And(x=w275, y=w276) -> (x .and. y?=w268:bool)
                n248 = property class="Bool"(reference=w269, "Value"=w268) -> ()  [unwired: 1 in, 2 out]
                n249 = Bundle By Name(cluster=errorcluster {"status"=FALSE, "code"=0, "source"=""} ("错误常量"), "status"=w268, "code"=w267) -> (w273:errorcluster)
                n250 = case shown="假" w274 {
                  tunnel: w273 -> [w282 _]
                  frame False {
                    n251 = call "报警处理.vi"("错误常量"=w282) -> ()  [unwired: 9 in, 2 out]
                  }
                  frame True {
                  }
                }
              }
            }
          }
          event User Event {
            n252 = event-data() -> ("试验项目"=w283:T1)  [unwired: 1 in]
            "试验项目" <- w283
            n253 = disable-structure shown="禁用" {
              disable-tunnel: w283 -> [w284 _]
              frame Disabled {
                n254 = global read "A180648.vi" "检测结果"() -> (w287:string[][][])
                n255 = global read "Global.vi" "Result"() -> (w285:refnum<vi>)
                n256 = Index Array(array=w287, index (dim 0)=w284) -> (element=w286:string[][])  [unwired: 2 in]
                n257 = property class="Tbl"(reference=w285, "Value"=w286) -> ()  [unwired: 1 in, 2 out]
              }
              frame Enabled {
              }
            }
          }
          event "试验项目": Value Change {
            n258 = event-data() -> ("NewVal"=w288:T1)  [unwired: 1 in]
            n259 = disable-structure shown="禁用" {
              disable-tunnel: w288 -> [w292 _]
              frame Disabled {
                n260 = global read "A180648.vi" "检测结果"() -> (w291:string[][][])
                n261 = global read "Global.vi" "Result"() -> (w289:refnum<vi>)
                n262 = Index Array(array=w291, index (dim 0)=w292) -> (element=w290:string[][])  [unwired: 2 in]
                n263 = property class="Tbl"(reference=w289, "Value"=w290) -> ()  [unwired: 1 in, 2 out]
              }
              frame Enabled {
              }
            }
          }
          event "0°曲线", "侧铆曲线", "45°曲线", "压装曲线", "功能试验", "逆向空载试验", "磨合": Scale Range Change {
            n264 = event-data() -> ("CtlRef"=w294:refnum<vi>)  [unwired: 1 in, 4 out]
            n265 = global read "Global.vi" "产品型号"() -> (w293:string)
            n266 = call "XY_conf.vi"("方式"=enum16{"写入", "读取"}."写入", "产品"=w293, "XY图引用"=w294) -> ()  [unwired: 4 in, 1 out]
          }
          event User Event {
            n267 = event-data() -> ("产品"=w298:string)  [unwired: 1 in]
            n268 = control-ref of="0°曲线"() -> (w297:refnum<vi>)
            n269 = control-ref of="压装曲线"() -> (w300:refnum<vi>)
            n270 = control-ref of="45°曲线"() -> (w296:refnum<vi>)
            n271 = control-ref of="侧铆曲线"() -> (w302:refnum<vi>)
            n272 = control-ref of="力特性试验"() -> (w301:refnum<vi>)
            n273 = Build Array(w297, w300, w296, w302, w301) -> (w299:refnum<vi>[])
            n274 = for {
              tunnel: w299 -> [w304] mode=indexing
              tunnel: w298 -> [w303]
              n275 = call "XY_conf.vi"("方式"=enum16{"写入", "读取"}."读取", "产品"=w303, "XY图引用"=w304) -> ()  [unwired: 4 in, 1 out]
            }
          }
          event Panel Close {
            n276 = event-data() -> ()  [unwired: 1 in, 4 out]
            n277 = global write "Global.vi" "程序关闭"(TRUE ("程序关闭")) -> ()
          }
          event "磨合": Mouse Enter; "磨合": Mouse Leave; "磨合": Mouse Move {
            n278 = event-data() -> ("CtlRef"=w309:refnum<vi>, "Type"=w307:T7)  [unwired: 1 in]
            n279 = call "CursorShow.vi"("nameShow"=TRUE, "Type"=w307, "Graph"=w309) -> ()  [unwired: 7 in, 2 out]
          }
          event "0°曲线", "侧铆曲线", "45°曲线", "压装曲线", "功能试验", "逆向空载试验", "磨合": Mouse Down {
            n280 = event-data() -> ("CtlRef"=w314:refnum<vi>, "Coords"=w313:T8, "Type"=w311:T7)  [unwired: 1 in]
            n281 = invoke class="XYGraph (严格)" method="Map Coords To XY"(reference=w314, "Coords"=w313) -> (reference out=w312:refnum<vi>, "XY"=w310:cluster{"X":dbl, "Y":dbl})  [unwired: 5 in, 5 out]
            n282 = call "CursorShow.vi"("游标.游标位置"=w310, "Type"=w311, "Graph"=w312) -> ()  [unwired: 7 in, 2 out]
          }
        }
        n283 = global read "Global.vi" "程序关闭"() -> (w263:bool)
      }
    }
  }
  n284 = Unregister For Events(event registration refnum=w5) -> ()  [unwired: 1 in, 1 out]
